vi "디버깅 실습(프로브).vi"() -> ()   [LabVIEW 2020]
panel:
  out "x+y":dbl
  out "숫자형 3":i32
  in  "숫자형 2":dbl
  in  "숫자형":dbl
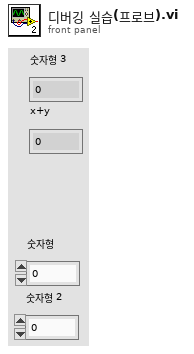
[diagram p1: front panel]
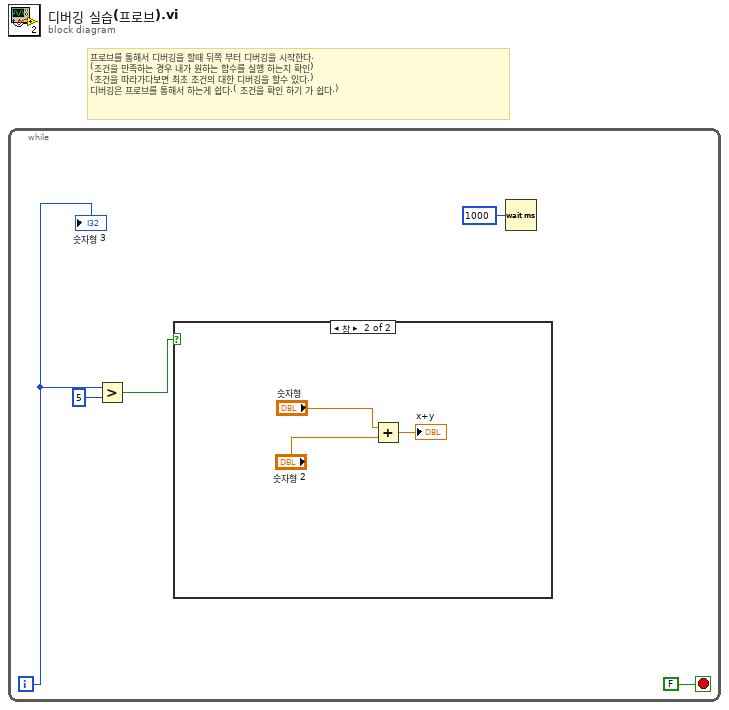
[diagram p0: block diagram]
diagram:
  # "프로브를 통해서 디버깅을 할때 뒤쪽 부터 디버깅을 시작한다.\n(조건을 만족하는 경우 내가 원하는 함수를 실행 하는지 확인)\n(조건을 따라가다보면 최초 조건의 대한 디버깅을 할수 있다.)\n디버깅은 프로브를 통해서 하는게 쉽다.( 조건을 확인 하기 가 쉽다.)"
  n1 = while {
    i -> [w5]
    stop <- FALSE stop-if-true
    n2 = Greater?(x=w5, y=5) -> (0:w3:bool)
    n3 = case shown="참" w3 {
      frame False {
      }
      frame True {
        n4 = Add(x="숫자형", y="숫자형 2") -> (x+y=→"x+y":dbl)
      }
    }
    n5 = Wait (ms)(milliseconds to wait=u32 1000 ("대기 시간 (ms)")) -> ()  [unwired: 1 out]
    "숫자형 3" <- w5
  }
